vi "Get FPGA Ref as Var.vi"(8 "error in (no error)":errorcluster, 11 "starter kit FPGA host in":refnum<class "NI_Robotics_Starter Kit Host_FPGA_2.0.lvclass">) -> (0 "error out":errorcluster, 2 "FPGA ref":variant, 3 "starter kit FPGA host out":refnum<class "NI_Robotics_Starter Kit Host_FPGA_2.0.lvclass">)   [LabVIEW 2017, in "NI_Robotics_Starter Kit Host_FPGA_2.0.lvclass"]
uses:
  <vilib>/robotics/Starter Kit/2.0/FPGA Host Interface/NI_Robotics_Starter Kit Host_FPGA_2.0.lvclass
  <vilib>/robotics/Starter Kit/2.0/FPGA Host Interface/NI_Robotics_Starter Kit Host_FPGA_2.0.lvclass/NI_Robotics_Starter Kit Host_FPGA_2.0.ctl
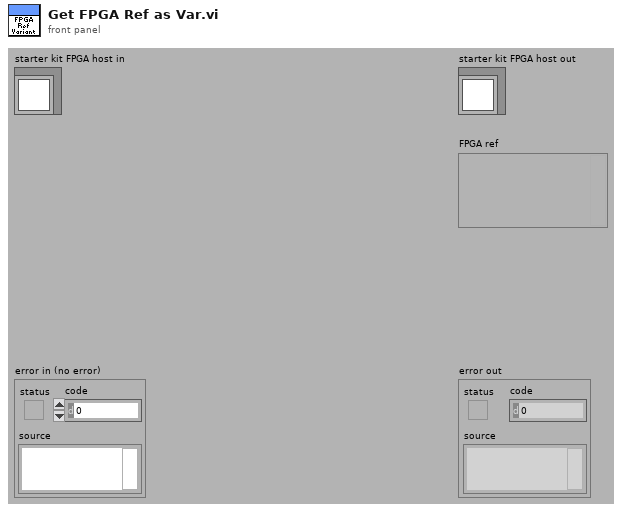
[diagram p1: front panel]
types:
  T1 = typedef "NI_Robotics_Starter Kit Host_FPGA_2.0.lvclass/FPGA Refnum.ctl" = refnum<k20>
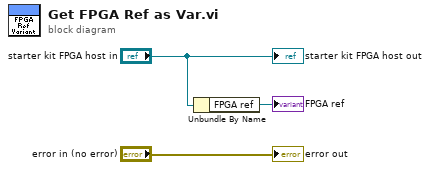
[diagram p0: block diagram]
diagram:
  n1 = Unbundle By Name("starter kit FPGA host in") -> ("FPGA ref"=→"FPGA ref":T1)
  "error out" <- "error in (no error)"
  "starter kit FPGA host out" <- "starter kit FPGA host in"
